vi "Measured Parameters.vi"(0 "VISA resource name":refnum<visa-resource-name>, 11 "error in (no error)":errorcluster) -> (2 "Dx":dbl format="%^.2e", 3 "Qx":dbl format="%^.2e", 4 "VISA resource name out":refnum<visa-resource-name>, 6 "Z":dbl format="%^.2e", 8 "Cx":dbl format="%^.2e", 10 "Rp":dbl format="%^.2e", 15 "error out":errorcluster)   [LabVIEW 2015, in "Agilent 428X Series.lvlib"]
doc: "This VI is to read the required parameter from the instrument in order to perform accuracy calculation."
uses:
  Agilent 428X Series.lvlib
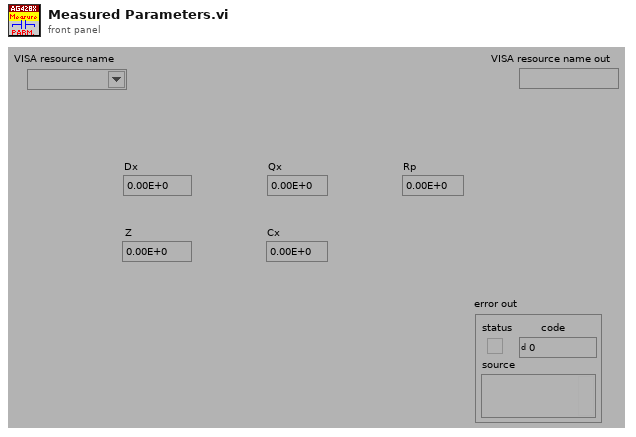
[diagram p1: front panel]
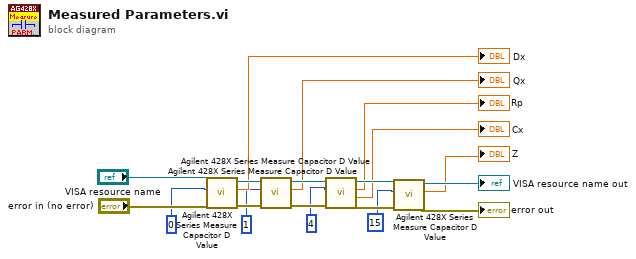
[diagram p0: block diagram]
diagram:
  n1 = call "Agilent 428X Series Measure Capacitor D Value.vi"("error in (no error)"="error in (no error)", "Imp Type (0: CPD)"=u32 0, "VISA resource name"="VISA resource name") -> ("error out"=w14:errorcluster, "Primary Value"=→"Dx":dbl, "VISA resource name out"=w15:refnum<visa-resource-name>)  [unwired: 4 in, 2 out]
  n2 = call "Agilent 428X Series Measure Capacitor D Value.vi"("error in (no error)"=w14, "Imp Type (0: CPD)"=u32 1, "VISA resource name"=w15) -> ("error out"=w16:errorcluster, "Primary Value"=→"Qx":dbl, "VISA resource name out"=w17:refnum<visa-resource-name>)  [unwired: 4 in, 2 out]
  n3 = call "Agilent 428X Series Measure Capacitor D Value.vi"("error in (no error)"=w16, "Imp Type (0: CPD)"=u32 4, "VISA resource name"=w17) -> ("error out"=w18:errorcluster, "Secondary Value"=→"Cx":dbl, "Primary Value"=→"Rp":dbl, "VISA resource name out"=w19:refnum<visa-resource-name>)  [unwired: 4 in, 1 out]
  n4 = call "Agilent 428X Series Measure Capacitor D Value.vi"("error in (no error)"=w18, "Imp Type (0: CPD)"=u32 15, "VISA resource name"=w19) -> ("error out"=→"error out":errorcluster, "Primary Value"=→"Z":dbl, "VISA resource name out"=→"VISA resource name out":refnum<visa-resource-name>)  [unwired: 4 in, 2 out]
